vi "Filter Instruments.vi"(10 "Ignore instruments":string[](array[string]), 11 "Instruments in":refnum<visa-resource-name>[](array[refnum])) -> (3 "Instruments out":refnum<visa-resource-name>[](array[refnum]))   [LabVIEW 2021]
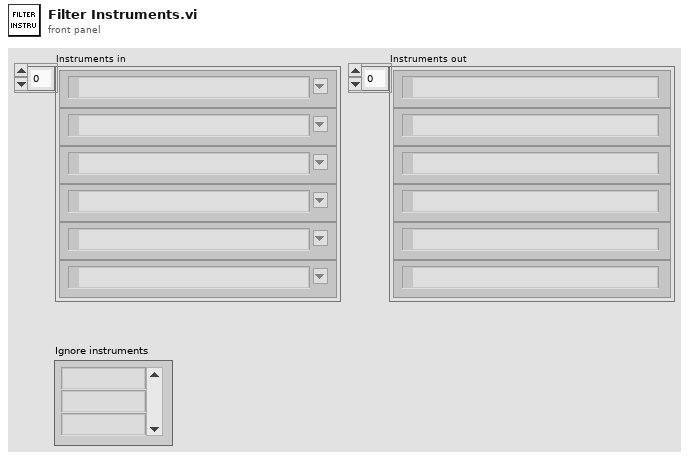
[diagram p1: front panel]
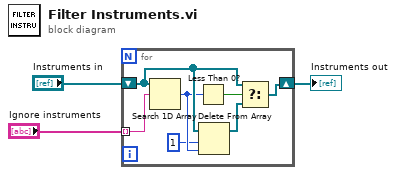
[diagram p0: block diagram]
diagram:
  n1 = for {
    tunnel: "Ignore instruments" -> [w10] mode=indexing
    shift-right: [w4] -> w1
    shift-left: "Instruments in" -> [w8]
    n2 = Search 1D Array(1D array=w8, element=w10) -> (index of element=w7:i32)  [unwired: 1 in]
    n3 = Less Than 0?(x=w7) -> (x < 0?=w9:bool)
    n4 = Delete From Array(array=w8, length=1, index=w7) -> (array with subset deleted=w5:refnum<visa-resource-name>[])  [unwired: 1 out]
    n5 = Select(t=w8, s=w9, f=w5) -> (s? t:f=w4:refnum<visa-resource-name>[])
  }
  "Instruments out" <- w1
